vi "WM Significant Wave Period.vi"(1 "Sampling Rate":dbl format="%.2f", 2 "Time Series":dbl[](array[numeric]) format="%.2f") -> (0 "Significant Wave Period":dbl format="%.2f")   [LabVIEW 2012]
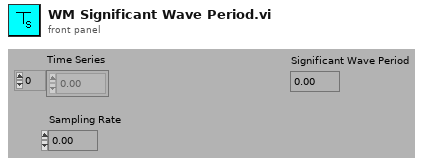
[diagram p1: front panel]
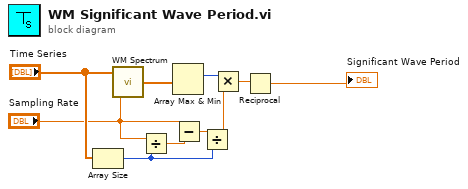
[diagram p0: block diagram]
diagram:
  n1 = Array Size(array="Time Series") -> (size(s)=w3:i32)
  n2 = call "WM Spectrum.vi"("Sampling Rate"="Sampling Rate", "Time Series"="Time Series") -> ("Spectra"=w9:dbl[])
  n3 = Divide(x="Sampling Rate", y=w3) -> (x/y=w5:dbl)
  n4 = Array Max & Min(array=w9) -> (max index (indices)=w8:i32)  [unwired: 3 out]
  n5 = Subtract(x="Sampling Rate", y=w5) -> (x-y=w4:dbl)
  n6 = Divide(x=w4, y=w3) -> (x/y=w2:dbl)
  n7 = Multiply(x=w8, y=w2) -> (x*y=w10:dbl)
  n8 = Reciprocal(x=w10) -> (1/x=→"Significant Wave Period":dbl)
